vi "Enque_Message_FGV.vi"(6 "Priority":bool, 8 "error in (no error)":errorcluster, 9 "Message Data":variant, 10 "Message":string, 11 "queue in":refnum<queue>) -> (0 "error out":errorcluster)   [LabVIEW 2024, in "SSL_Certification.lvlib"]
doc: "ThisVI\n------------------------------\nEnqueue Message\n------------------------------\n-Enqueue the message in message queue.\n-set Priority to true to enqueue at oposite end"
uses:
  SSL_Certification.lvlib
  PrivateControls/FGV_Queue_Control.ctl
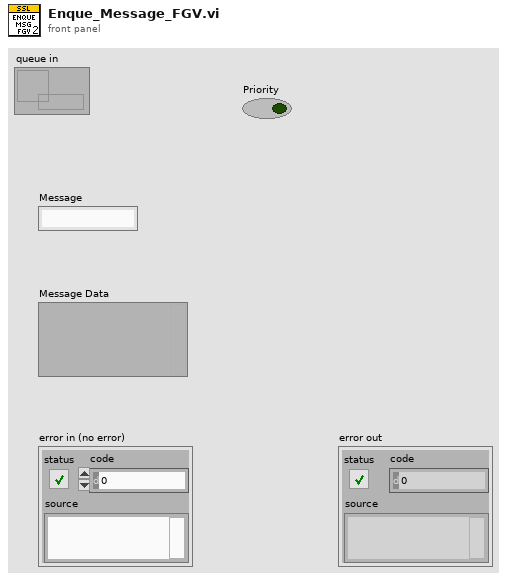
[diagram p1: front panel]
types:
  T1 = cluster{"Message":string, "Message Data":variant}
  T2 = typedef "SSL_Certification.lvlib/FGV_Queue_Control.ctl" = enum16{"Release", "Get", "Set"}
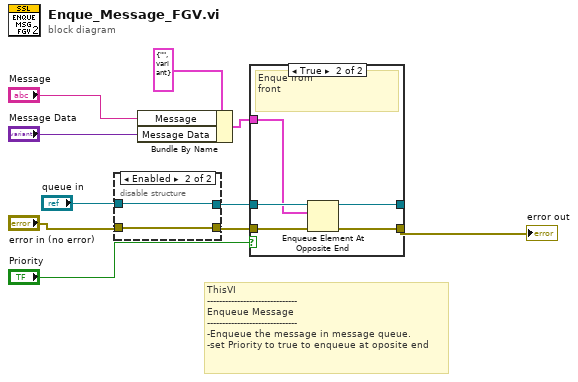
[diagram p0: block diagram]
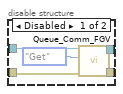
[diagram p2: hidden frame]
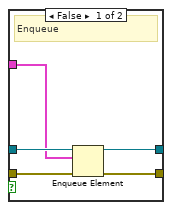
[diagram p3: hidden frame]
diagram:
  # "ThisVI\n------------------------------\nEnqueue Message\n------------------------------\n-Enqueue the message in message queue.\n-set Priority to true to enqueue at oposite end"
  n1 = disable-structure shown="Enabled" {
    disable-tunnel: [w15 w17] -> w6
    disable-tunnel: [w14 w16] -> w4
    disable-tunnel: "error in (no error)" -> [w12 w16]
    disable-tunnel: "queue in" -> [w11 w17]
    frame Disabled {
      n2 = call "Queue_Comm_FGV.vi"("error in (no error)"=w12, "Enum"=FGV_Queue_Control."Get", "queue in"=w11) -> ("error Out"=w14:errorcluster, "queue Out"=w15:refnum<queue>)  [unwired: 7 in]
    }
    frame Enabled {
    }
  }
  n3 = Bundle By Name(cluster=T1 {"Message"="", "Message Data"=variant} ("element"), "Message"="Message", "Message Data"="Message Data") -> (w8:T1)
  n4 = case shown="True" "Priority" {
    tunnel: w4 -> [w22 w27]
    tunnel: [w21 w26] -> w5
    tunnel: w6 -> [w19 w25]
    tunnel: [w20 w24] -> _
    tunnel: w8 -> [w18 w23]
    frame False {
      # "Enqueue"
      n5 = Enqueue Element(queue=w19, element=w18, error in (no error)=w22) -> (queue out=w20:refnum<queue>, error out=w21:errorcluster)  [unwired: 1 in, 1 out]
    }
    frame True {
      # "Enque from\nfront"
      n6 = Enqueue Element At Opposite End(queue=w25, element=w23, error in (no error)=w27) -> (queue out=w24:refnum<queue>, error out=w26:errorcluster)  [unwired: 1 in, 1 out]
    }
  }
  "error out" <- w5
